vi "Datacut(ver15).vi"(0 "Input Total P":i32[](array[numeric]), 1 "moveLog(Row, Col.)入力":i32[][][](array[numeric]), 2 "Input 1st or 2nd":string[](array[string])) -> (3 "moveLog(Row, Col.)出力":i32[][][](array[numeric]), 4 "Output Total P":i32[](array[numeric]), 5 "delete coount":i32, 6 "Input 1st or 2nd 2":string[](array[string]))   [LabVIEW 2016]
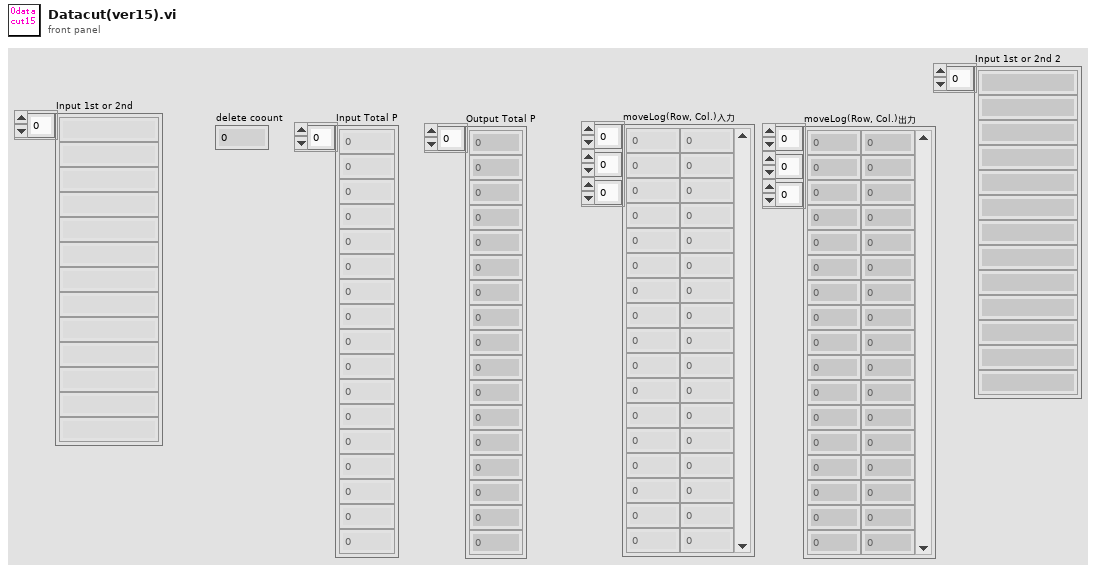
[diagram p1: front panel]
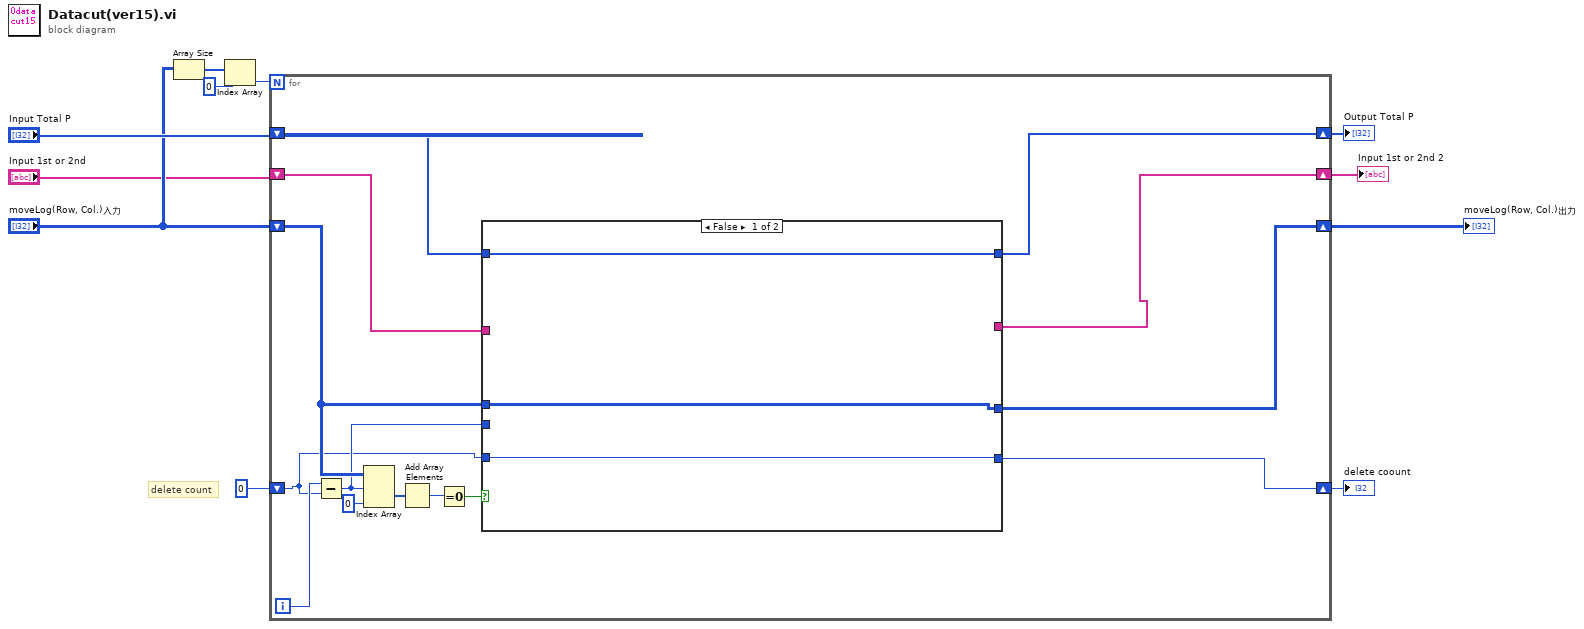
[diagram p0: block diagram]
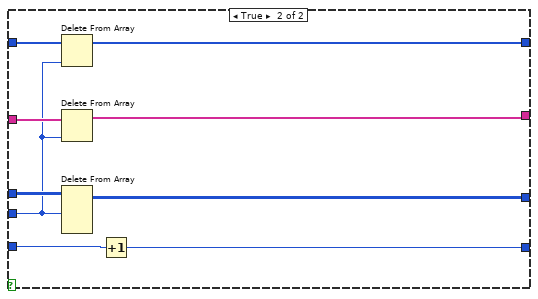
[diagram p2: hidden frame]
diagram:
  # "delete count"
  n1 = Array Size(array="moveLog(Row, Col.)入力") -> (size(s)=w7:i32[])
  n2 = Index Array(array=w7, index=0 ("指標")) -> (element=w5:i32)
  n3 = for {
    N: w5 -> [_]
    shift-right: [w19] -> w10
    shift-left: "moveLog(Row, Col.)入力" -> [w20]
    shift-right: [w16] -> w3
    shift-left: "Input Total P" -> [w17]
    shift-right: [w14] -> w4
    shift-left: 0 -> [w15]
    shift-right: [w12] -> w1
    shift-left: "Input 1st or 2nd" -> [w13]
    i -> [w25]
    n4 = Subtract(x=w25, y=w15) -> (x-y=w18:i32)
    n5 = Index Array(array=w20, index (dim 0)=w18, index (dim 2)=0 ("無効な指標 （列）")) -> (element=w23:i32[])  [unwired: 1 in]
    n6 = Add Array Elements(numeric array=w23) -> (sum=w22:i32)
    n7 = Equal To 0?(x=w22) -> (x = 0?=w21:bool)
    n8 = case shown="False" w21 {
      tunnel: w20 -> [w27 w37]
      tunnel: w18 -> [_ w30]
      tunnel: [w27 w36] -> w19
      tunnel: w17 -> [w28 w35]
      tunnel: [w28 w34] -> w16
      tunnel: w15 -> [w26 w33]
      tunnel: [w26 w32] -> w14
      tunnel: w13 -> [_ w31]
      tunnel: [_ w29] -> w12
      frame False {
      }
      frame True {
        n9 = Delete From Array(array=w35, index=w30) -> (array with subset deleted=w34:i32[])  [unwired: 1 in, 1 out]
        n10 = Delete From Array(array=w31, index=w30) -> (array with subset deleted=w29:string[])  [unwired: 1 in, 1 out]
        n11 = Delete From Array(array=w37, index (dim 0)=w30) -> (array with subset deleted=w36:i32[][][])  [unwired: 3 in, 1 out]
        n12 = Increment(x=w33) -> (x+1=w32:i32)
      }
    }
  }
  "moveLog(Row, Col.)出力" <- w10
  "delete coount" <- w4
  "Output Total P" <- w3
  "Input 1st or 2nd 2" <- w1
